vi "GLBL_AI.vi"(9 "analog in 0_15":T1, 10 "write_read":bool) -> (1 "analog out":T1)   [LabVIEW 2020]
uses:
  controls/AI_0_15.ctl
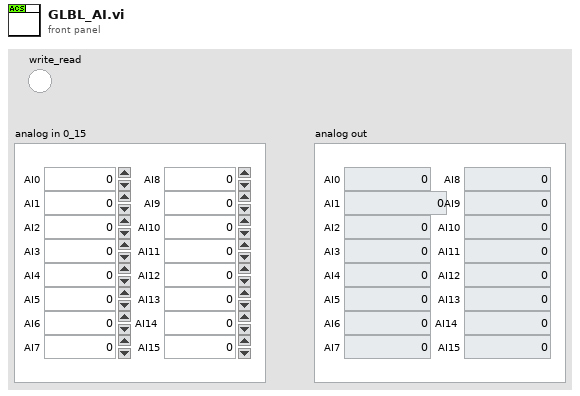
[diagram p1: front panel]
types:
  T1 = typedef "AI_0_15.ctl" = cluster{"AI0":dbl, "AI1":dbl, "AI2":dbl, "AI3":dbl, "AI4":dbl, "AI5":dbl, "AI6":dbl, "AI7":dbl, "AI8":dbl, "AI9":dbl, "AI10":dbl, "AI11":dbl, "AI12":dbl, "AI13":dbl, "AI14":dbl, "AI15":dbl}
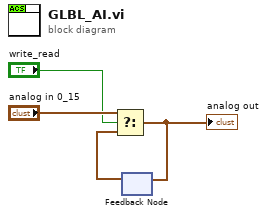
[diagram p0: block diagram]
diagram:
  n1 = feedback #1() -> (w3:T1)  [unwired: 1 in]
  n2 = Select(t="analog in 0_15", s="write_read", f=w3) -> (s? t:f=w2:T1)
  "analog out" <- w2
  n3 = feedback-in #1(w2) -> ()
